vi "RunsDialog.vi"(8 "Error In":errorcluster, 11 "Runs In":T1[](array[typedef])) -> (0 "Error Out":errorcluster)   [LabVIEW 2012]
uses:
  DisplayRun.ctl
  ExperimentRun.ctl
  ExperimentRunTiming.ctl
  ExperimentRunDose.ctl
  ExperimentRunFluence.ctl
  ExperimentRunTotalCharge.ctl
  libs/LV-Utilities/LV-Utilities.lvlib
panel:
  in  "CLOSE":bool
  out "Display Runs":T6[](array[typedef]) {"Stop Current" format="%.3p"; "Start Current" format="%.3p"; "Stop Fluence" format="%.3e"; "Start Fluence" format="%.3e"; "Stop Dose" format="%.3e"; "Start Dose" format="%.3e"; "Stop Time" format="%<%H:%M:%S\n%m/%d/%Y>T"; "Start Time" format="%<%H:%M:%S\n%m/%d/%Y>T"}
  # "Current"
  # "Stop"
  # "Start"
  # "Fluence"
  # "Stop"
  # "Start"
  # "Dose"
  # "Stop"
  # "Start"
  # "Timing"
  # "Stop"
  # "Start"
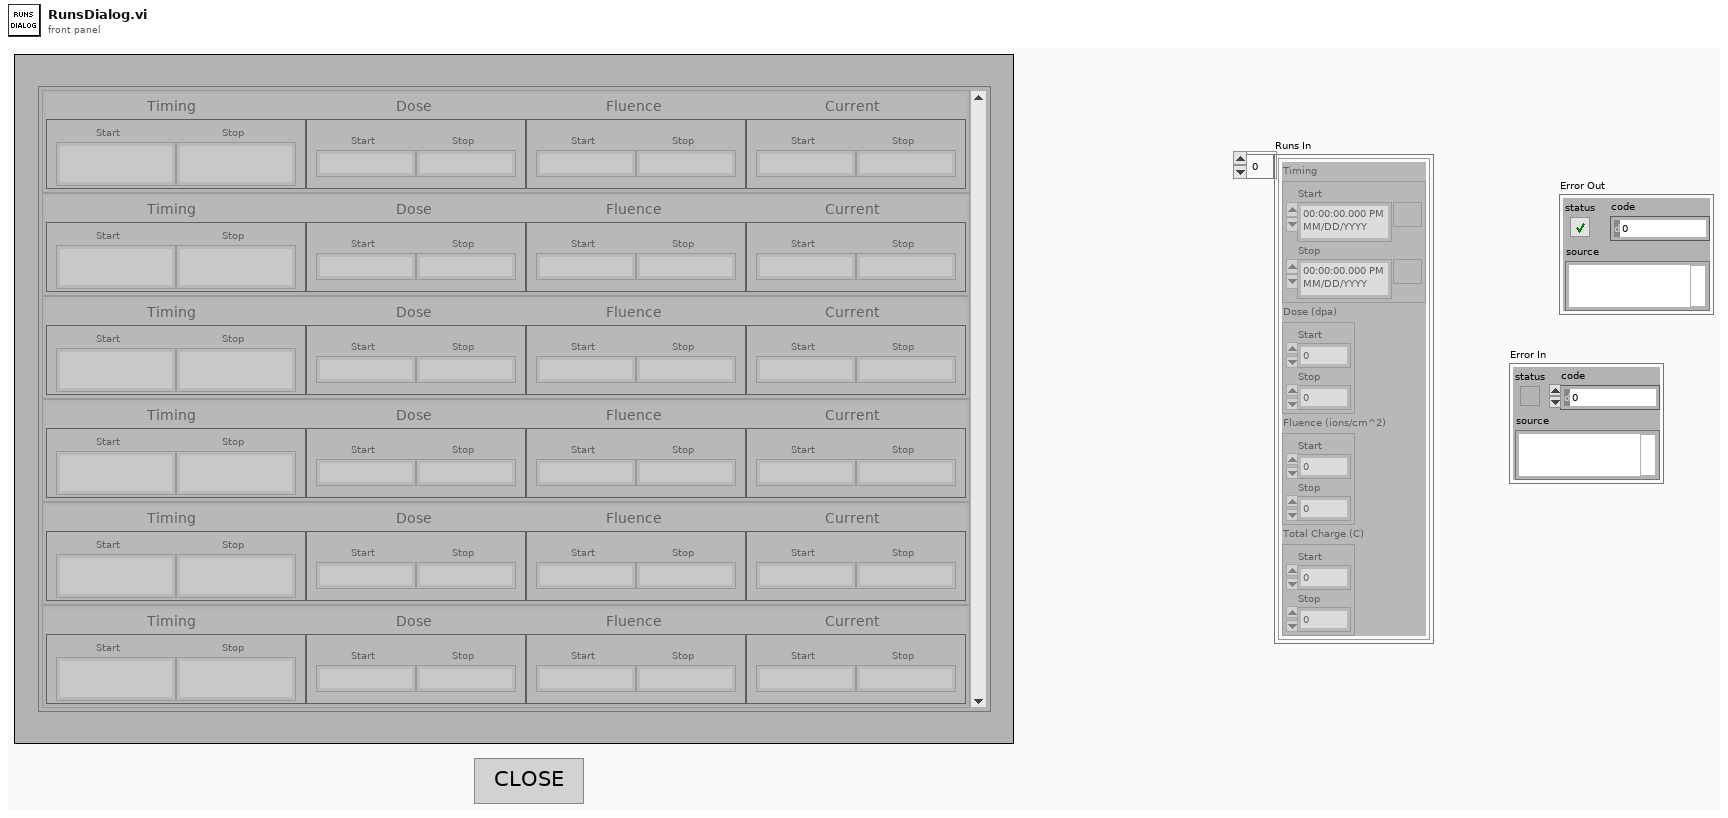
[diagram p1: front panel]
types:
  T1 = typedef "ExperimentRun.ctl" = cluster{"Timing":T2, "Dose (dpa)":T3, "Fluence (ions/cm^2)":T4, "Total Charge (C)":T5}
  T2 = typedef "ExperimentRunTiming.ctl" = cluster{"Start":timestamp, "Stop":timestamp}
  T3 = typedef "ExperimentRunDose.ctl" = cluster{"Start":dbl, "Stop":dbl}
  T4 = typedef "ExperimentRunFluence.ctl" = cluster{"Start":dbl, "Stop":dbl}
  T5 = typedef "ExperimentRunTotalCharge.ctl" = cluster{"Start":dbl, "Stop":dbl}
  T6 = typedef "DisplayRun.ctl" = cluster{"Start Time":timestamp, "Stop Time":timestamp, "Start Dose":dbl, "Stop Dose":dbl, "Start Fluence":dbl, "Stop Fluence":dbl, "Start Current":dbl, "Stop Current":dbl}
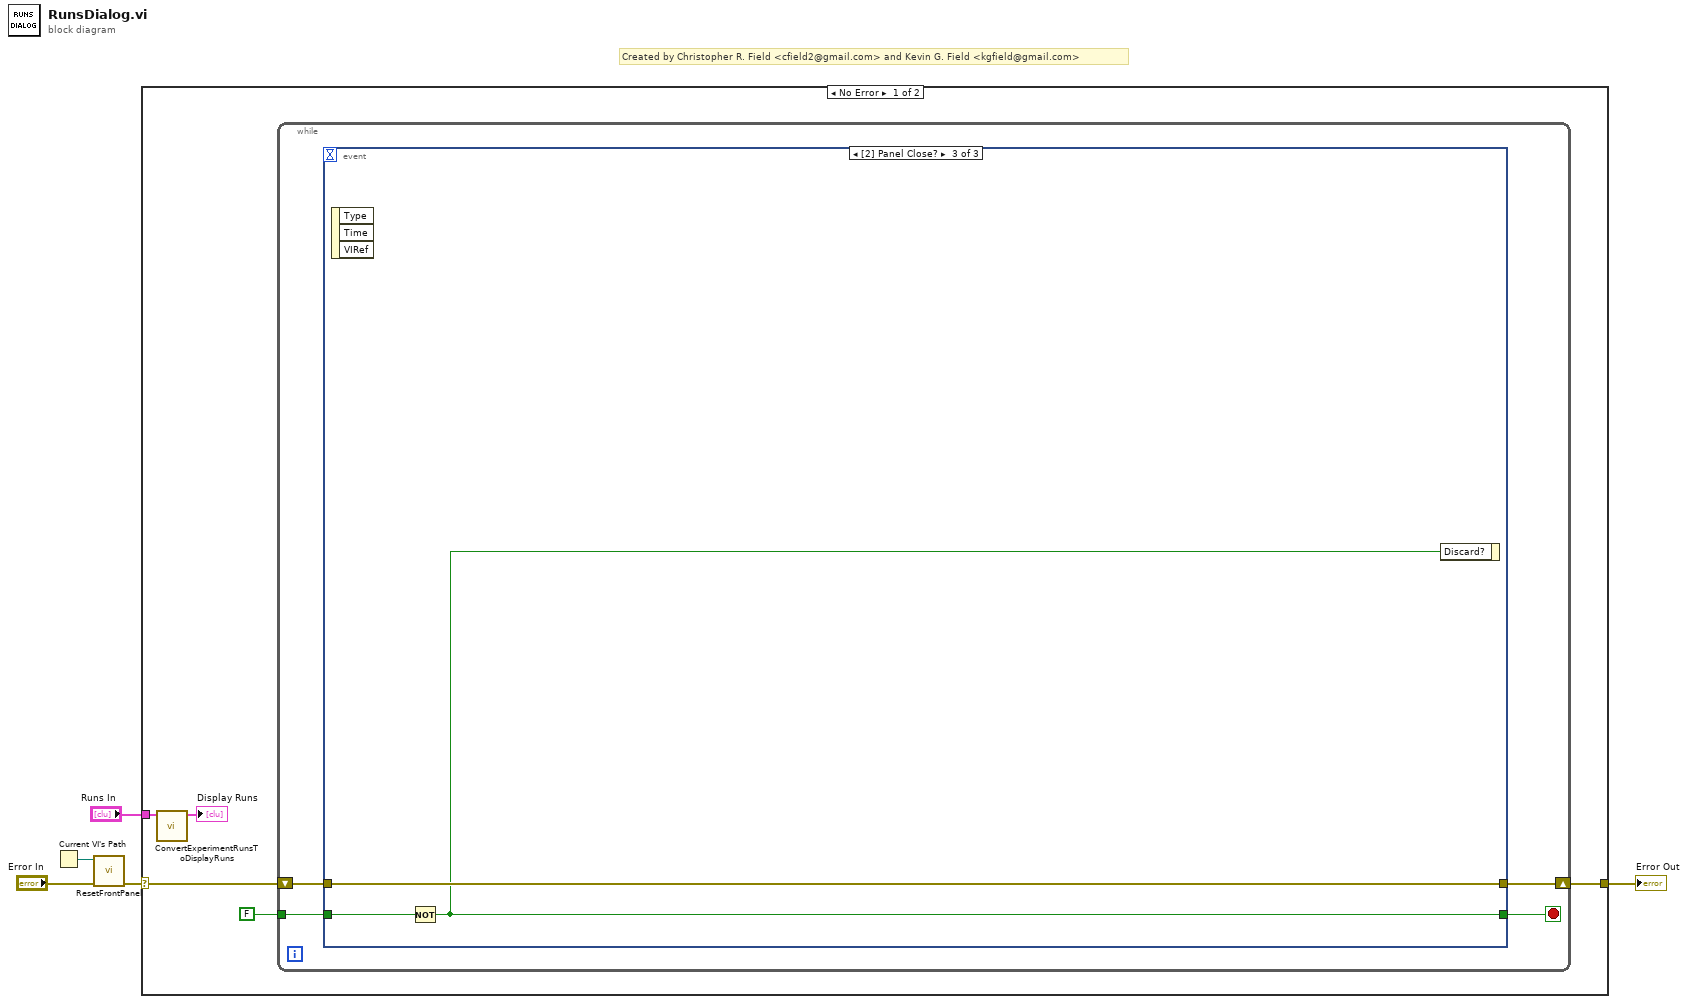
[diagram p0: block diagram]
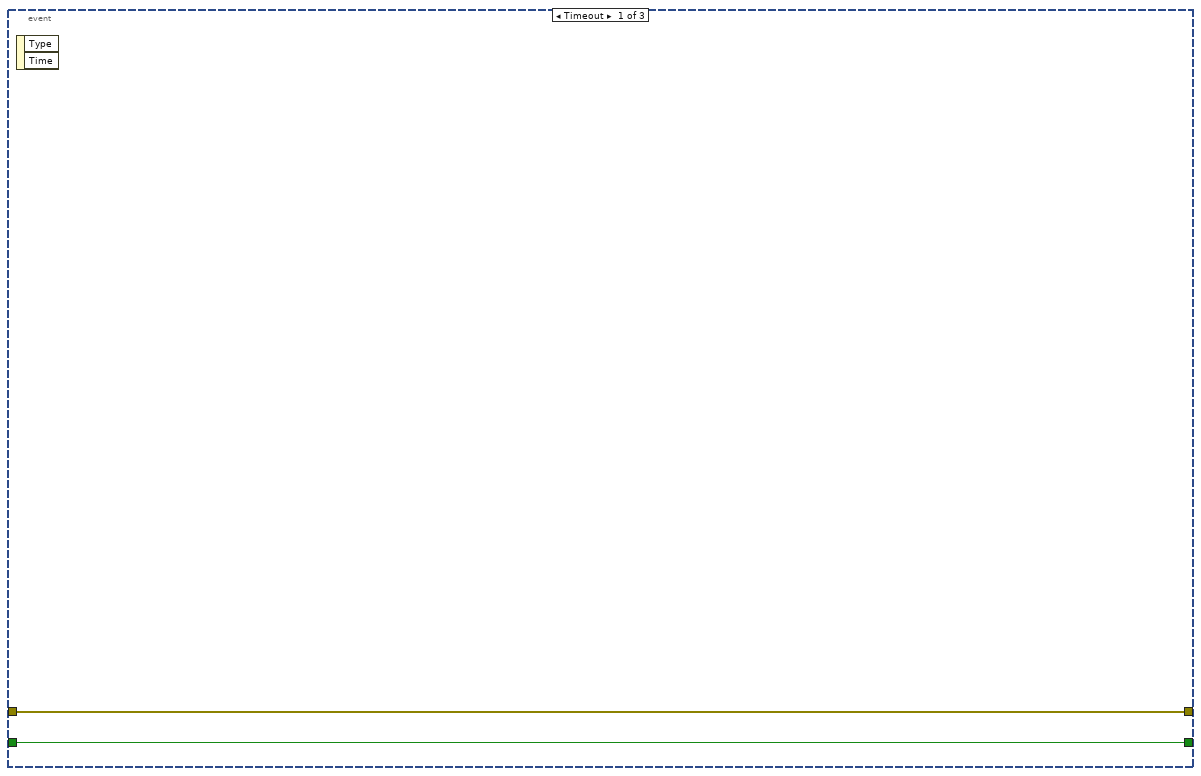
[diagram p2: hidden frame]
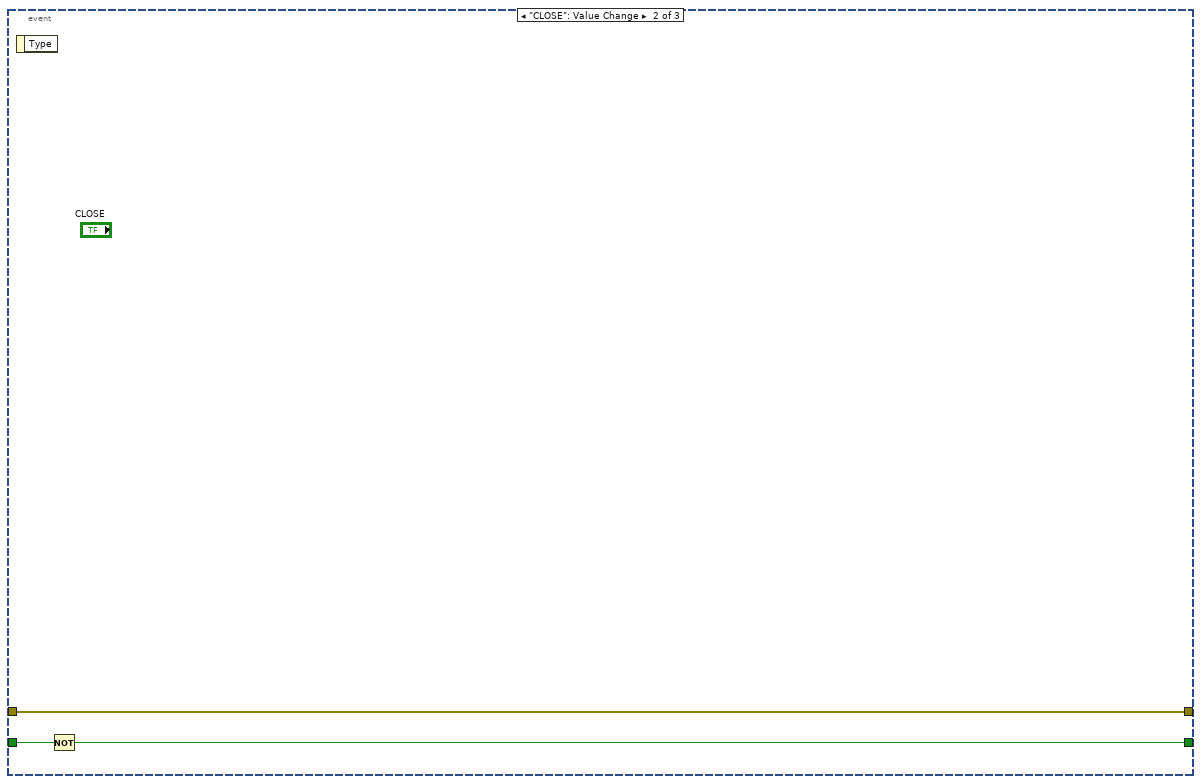
[diagram p3: hidden frame]
diagram:
  # "Created by Christopher R. Field <cfield2@gmail.com> and Kevin G. Field <kgfield@gmail.com>"
  n1 = Current VI's Path() -> (path=w5:path)
  n2 = call "ResetFrontPanel.vi"("Error In"="Error In", "VI Path"=w5) -> ("Error Out"=w1:errorcluster)  [unwired: 9 in]
  n3 = case shown="No Error" w1 {
    selector: w1 -> [w6 w23]
    tunnel: [w9 w23] -> w3
    tunnel: "Runs In" -> [w7 _]
    frame No Error {
      n4 = call "ConvertExperimentRunsToDisplayRuns.vi"("Experiment Runs"=w7) -> ("Display Runs"=→"Display Runs":T6[])  [unwired: 10 in]
      n5 = while {
        tunnel: FALSE -> [w13]
        shift-right: [w11] -> w9
        shift-left: w6 -> [w14]
        stop <- w12 stop-if-true
        n6 = event shown="[2] Panel Close?" {
          selector: _ -> [_ _ _]
          dyn-events: _ -> [_ _ _]
          timeout: _ -> [_ _ _]
          tunnel: w13 -> [w16 w19 w22]
          tunnel: [w16 w18 w20] -> w12
          tunnel: w14 -> [w15 w17 w21]
          tunnel: [w15 w17 w21] -> w11
          event Timeout {
            n7 = event-data() -> ()  [unwired: 1 in, 2 out]
          }
          event "CLOSE": Value Change {
            n8 = event-data() -> ()  [unwired: 1 in, 1 out]
            n9 = Not(x=w19) -> (.not. x?=w18:bool)
          }
          event Panel Close? {
            n10 = event-data() -> ()  [unwired: 1 in, 3 out]
            n11 = Not(x=w22) -> (.not. x?=w20:bool)
            n12 = event-data("Discard?"=w20) -> ()  [unwired: 1 in, 1 out]
          }
        }
      }
    }
    frame Error {
    }
  }
  "Error Out" <- w3
